vi "dfd_NStage MRate Get Filter Gain.vi"(11 "multirate filters":T1[](array[typedef]) {"mMRate_SumWl" min=1 max=32 step=1; "mMRate_InputIwl" min=1 max=32 step=1; "mMRate_GainWl" min=1 max=32 step=1; "mMRate_OutputWl" min=1 max=32 step=1; "mMRate_InputWl" min=1 max=32 step=1; "mMRate_CoefWl" min=1 max=32 step=1; "mMRate_Mode" items=["Default"=-1, "No Rate Change"=0, "Interpolation"=1, "Decimation"=2, "Interpolated"=3, "Rational"=4]}) -> (1 "gain":dbl, 2 "NStage output -fwl":i16)   [LabVIEW 2017, in "NI_DigFilter_FXP.lvlib"]
uses:
  <vilib>/addons/Digital Filter Design/NI_DigFilter_FXP.lvlib
  <vilib>/addons/Digital Filter Design/_Objects.llb/DFD Multirate Filter Obj.ctl
  <vilib>/addons/Digital Filter Design/_Objects.llb/DFD Multirate Mode.ctl
  <vilib>/addons/Digital Filter Design/_Objects.llb/DFD Coef Norm Type.ctl
  <vilib>/addons/Digital Filter Design/_Objects.llb/DFD Round-off Mode.ctl
  <vilib>/addons/Digital Filter Design/_Objects.llb/DFD FXP MRate Multiply Mode.ctl
  <vilib>/addons/Digital Filter Design/NI_DigFilterLicensed.lvlib
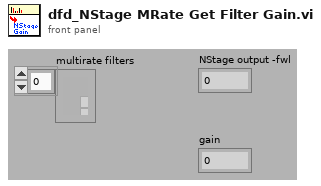
[diagram p1: front panel]
types:
  T1 = typedef "NI_DigFilterLicensed.lvlib/DFD Multirate Filter Obj.ctl" = cluster{"mMRate_Structure":enum16{"CIC", "FIR", "IIR", "Lattice"}, "mMRate_Mode":T2, "mMRate_Factor":i32, "mMRate_FIRParams":cluster{"mMRate_FIR_H":dbl[], "mMRate_FIR_IsNyquist?":bool, "mMRate_FIR_IsSymmetric?":bool}, "mMRate_CICParams":cluster{"mMRate_CIC_#Stage":i32, "mMRate_CIC_Lag":i32, "mMRate_CIC_Type":enum16{"Lowpass", "Highpass"}}, "mMRate_Order":i32, "mMRate_Version":string, "mMRate_Comments":string, "mMRate_RationalFactor":cluster{"mMRate_L":i32, "mMRate_M":i32}, "mMRate_Fs":dbl, "mMRate_Quantized?":bool, "mMRate_QFilterGain":dbl, "mMRate_CoefWl":i16, "mMRate_Scaling":cluster{"mMRate_ScaleByPowerOf2?":bool, "mMRate_ScaleType":T3}, "mMRate_InputWl":i16, "mMRate_OutputWl":i16, "mMRate_OutputMode":T4, "mMRate_MultMode":T5, "mMRate_BitPruning":bool, "mMRate_GainWl":i16, "mMRate_OutputFwl":i16, "mMRate_SumIwl":i16, "mMRate_InputIwl ":i16, "mMRate_SumWl":i16, "mMRate_CoefIwl":i16}
  T2 = typedef "NI_DigFilterLicensed.lvlib/DFD Multirate Mode.ctl" = i16
  T3 = typedef "NI_DigFilterLicensed.lvlib/DFD Coef Norm Type.ctl" = enum16{"No Norm", "Time Domain 1-Norm", "Time Domain 2-Norm", "Time Domain Inf-Norm"}
  T4 = typedef "NI_DigFilterLicensed.lvlib/DFD Round-off Mode.ctl" = enum16{"Nearest", "Truncation"}
  T5 = typedef "NI_DigFilterLicensed.lvlib/DFD FXP MRate Multiply Mode.ctl" = enum16{"Truncated", "Full"}
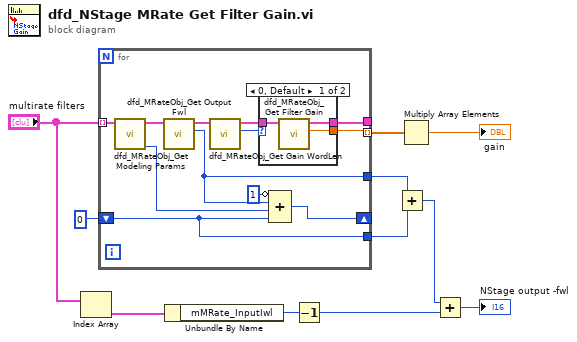
[diagram p0: block diagram]
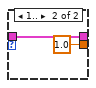
[diagram p2: hidden frame]
diagram:
  n1 = Index Array(array="multirate filters") -> (element=w5:T1)  [unwired: 1 in]
  n2 = for {
    tunnel: "multirate filters" -> [w20] mode=indexing
    tunnel: [w21] -> w10 mode=indexing
    shift-right: [w17] -> _
    shift-left: i16 0 -> [w14]
    tunnel: [w14] -> w7
    tunnel: [w13] -> _
    tunnel: [w12] -> w8
    n3 = call <vilib>:"dfd_MRateObj_Get Modeling Params.vi"("multirate filter in"=w20) -> ("output wl"=w16:i16, "dup multirate filter"=w19:T1)  [unwired: 9 out]
    n4 = call <vilib>:"dfd_MRateObj_Get Output Fwl.vi"("multirate filter in"=w19) -> ("output fwl"=w12:i16, "dup multirate filter"=w18:T1)  [unwired: 9 out]
    n5 = call <vilib>:"dfd_MRateObj_Get Gain WordLen.vi"("multirate filter in"=w18) -> ("gain wl"=w22:i16, "dup multirate filter"=w23:T1)  [unwired: 9 out]
    n6 = case shown="0, Default" w22 {
      tunnel: w23 -> [w26 w27]
      tunnel: [w25 1.0 ("gain")] -> w21
      tunnel: [w24 w27] -> w13
      frame 0, Default {
        n7 = call <vilib>:"dfd_MRateObj_Get Filter Gain.vi"("multirate filter in"=w26) -> ("gain"=w25:dbl, "dup multirate filter"=w24:T1)  [unwired: 9 out]
      }
      frame 1.. {
      }
    }
    n8 = Compound Arithmetic op=ADD(invert i16 1 ("value"), w12, w16, w14) -> (w17:i16)
  }
  n9 = Unbundle By Name(w5) -> ("mMRate_InputIwl"=w4:i16)
  n10 = Decrement(x=w4) -> (x-1=w2:i16)
  n11 = Add(x=w8, y=w7) -> (x+y=w3:i16)
  n12 = Multiply Array Elements(1:w10) -> (0:→"gain":dbl)
  n13 = Add(x=w3, y=w2) -> (x+y=→"NStage output -fwl":i16)
